vi "ShooterBones.vi"   [LabVIEW 2013]
uses:
  <vilib>/Rock Robotics/WPI/Solenoid/WPI_SolenoidOpenSingle.vi
  <vilib>/Rock Robotics/WPI/Solenoid/WPI_SolenoidOpenDouble.vi
types:
  T1 = typedef "WPI_SolenoidDevRef.ctl" = cluster{"DevStatus":errorcluster, "Solenoid Module":T2, "Forward Solenoid Channel":T3, "Reverse Solenoid Channel":T3}
  T2 = typedef "FPGA_TypedefSolenoidModule.ctl" = enum16{"Solenoid Module 1", "Solenoid Module 2"}
  T3 = typedef "WPI_SolenoidChannel.ctl" = enum8{"Solenoid 1", "Solenoid 2", "Solenoid 3", "Solenoid 4", "Solenoid 5", "Solenoid 6", "Solenoid 7", "Solenoid 8", "Invalid"}
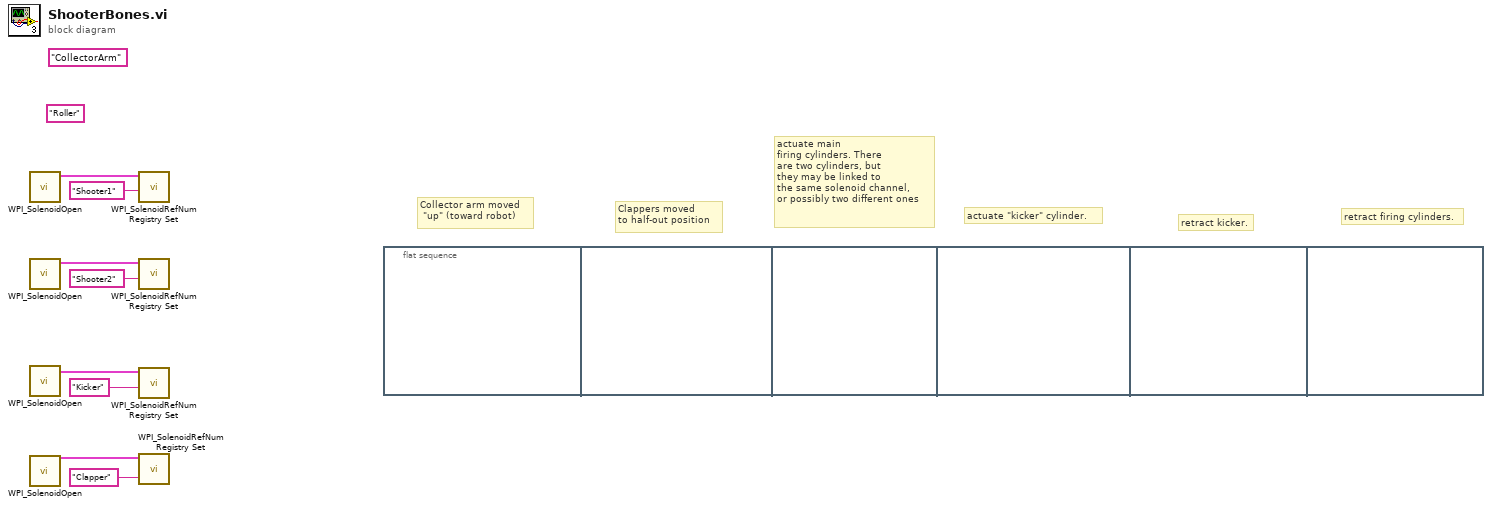
[diagram p0: block diagram]
diagram:
  (unwired) "Roller"
  (unwired) "CollectorArm"
  # "retract firing cylinders."
  # "retract kicker."
  # "actuate \"kicker\" cylinder."
  # "actuate main \nfiring cylinders. There \nare two cylinders, but \nthey may be linked to \nthe same solenoid channel, \nor possibly two different ones"
  # "Clappers moved\nto half-out position"
  # "Collector arm moved\n \"up\" (toward robot)"
  n1 = call-poly <vilib>:"WPI_SolenoidOpen.vi"() -> ("SolenoidDevRef"=w8:T1)  [unwired: 10 in, 1 out]
  n2 = call-poly <vilib>:"WPI_SolenoidOpen.vi"() -> ("SolenoidDevRef"=w3:T1)  [unwired: 10 in, 1 out]
  n3 = call-poly <vilib>:"WPI_SolenoidOpen.vi"() -> ("SolenoidDevRef"=w2:T1)  [unwired: 10 in, 1 out]
  n4 = call-poly <vilib>:"WPI_SolenoidOpen.vi"() -> ("SolenoidDevRef"=w1:T1)  [unwired: 10 in, 1 out]
  n5 = call <vilib>:"WPI_SolenoidRefNum Registry Set.vi"("refnum name"="Shooter1", "SolenoidDevRef"=w8) -> ()  [unwired: 8 in, 2 out]
  n6 = call <vilib>:"WPI_SolenoidRefNum Registry Set.vi"("refnum name"="Shooter2", "SolenoidDevRef"=w3) -> ()  [unwired: 8 in, 2 out]
  n7 = call <vilib>:"WPI_SolenoidRefNum Registry Set.vi"("refnum name"="Kicker", "SolenoidDevRef"=w2) -> ()  [unwired: 8 in, 2 out]
  n8 = call <vilib>:"WPI_SolenoidRefNum Registry Set.vi"("refnum name"="Clapper", "SolenoidDevRef"=w1) -> ()  [unwired: 8 in, 2 out]
  n9 = flat-sequence {
    frame #0 {
    }
    frame #1 {
    }
    frame #2 {
    }
    frame #3 {
    }
    frame #4 {
    }
    frame #5 {
    }
  }
